vi "Update.vi"(8 "error in (no error)":errorcluster, 9 "Audio Block 2":dbl[][](array[numeric]), 10 "Audio Block 1":dbl[][](array[numeric]), 11 "Mixer in":refnum<class "Mixer.lvclass">) -> (0 "error out":errorcluster, 1 "Headphones Audio Block Out":dbl[][](array[numeric]), 2 "Master Audio Block Out":dbl[][](array[numeric]), 3 "Mixer out":refnum<class "Mixer.lvclass">)   [LabVIEW 2018, in "Mixer.lvclass"]
uses:
  Mixer.lvclass
  Mixer.lvclass/Mixer.ctl
  Channel/Channel.lvclass
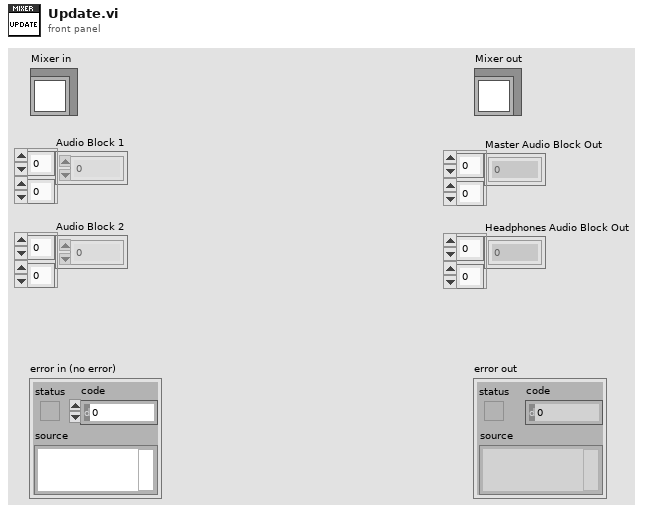
[diagram p1: front panel]
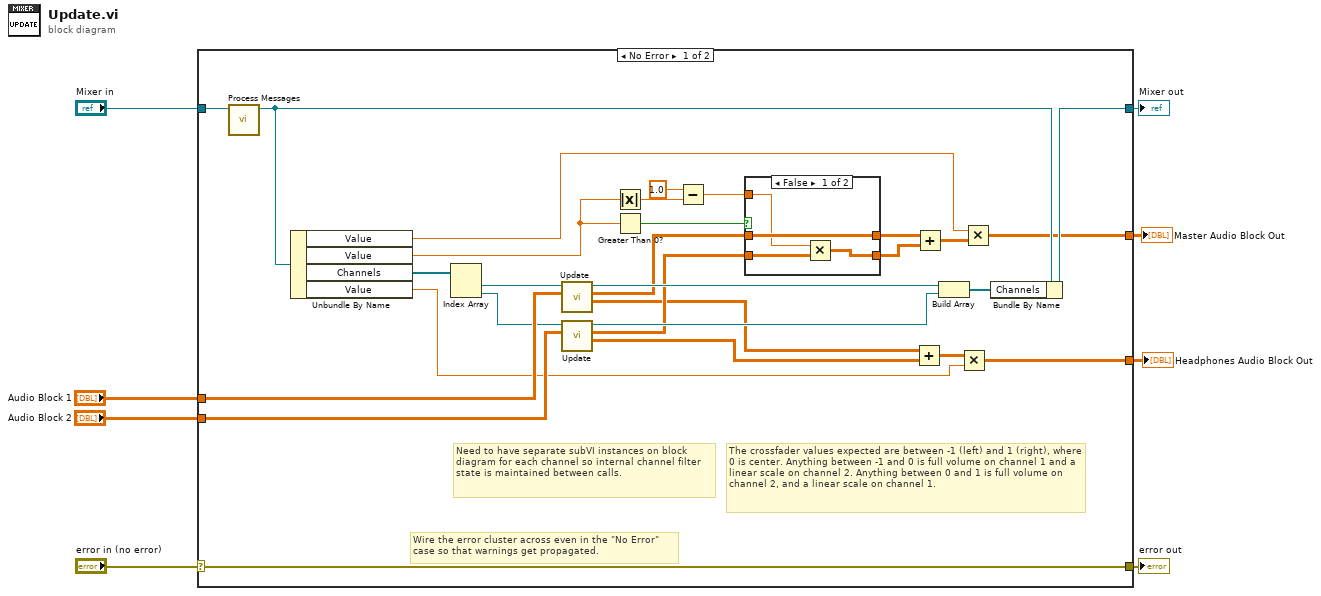
[diagram p0: block diagram]
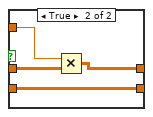
[diagram p2: hidden frame]
diagram:
  n1 = case shown="No Error" "error in (no error)" {
    selector: "error in (no error)" -> [w37 w48]
    tunnel: [w37 w48] -> w7
    tunnel: [w34 w47] -> w5
    tunnel: "Mixer in" -> [w36 w47]
    tunnel: "Audio Block 1" -> [w29 w46]
    tunnel: "Audio Block 2" -> [w28 _]
    tunnel: [w16 w46] -> w2
    tunnel: [w9 w46] -> w1
    frame No Error {
      # "Need to have separate subVI instances on block diagram for each channel so internal channel filter state is maintained between calls."
      # "The crossfader values expected are between -1 (left) and 1 (right), where 0 is center. Anything between -1 and 0 is full volume on channel 1 and a linear scale on channel 2. Anything between 0 and 1 is full volume on channel 2, and a linear scale on channel 1."
      # "Wire the error cluster across even in the \"No Error\"\ncase so that warnings get propagated."
      n2 = call "Process Messages.vi"("Mixer in"=w36) -> ("Mixer out"=w35:refnum<class "Mixer.lvclass">)  [unwired: 9 in, 1 out]
      n3 = Unbundle By Name(w35) -> ("Value"=w17:dbl, "Value"=w24:dbl, "Channels"=w33:refnum<class "Channel.lvclass">[], "Value"=w10:dbl)
      n4 = Index Array(array=w33) -> (element #1=w15:refnum<class "Channel.lvclass">, element #2=w14:refnum<class "Channel.lvclass">)  [unwired: 2 in]
      n5 = call "Update.vi"("Audio Block In"=w29, "Channel in"=w15) -> ("Headphones Audio Block Out"=w13:dbl[][], "Master Audio Block Out"=w26:dbl[][], "Channel out"=w32:refnum<class "Channel.lvclass">)  [unwired: 6 in, 1 out]
      n6 = call "Update.vi"("Audio Block In"=w28, "Channel in"=w14) -> ("Headphones Audio Block Out"=w12:dbl[][], "Master Audio Block Out"=w25:dbl[][], "Channel out"=w31:refnum<class "Channel.lvclass">)  [unwired: 6 in, 1 out]
      n7 = Absolute Value(x=w24) -> (abs(x)=w22:dbl)
      n8 = Greater Than 0?(x=w24) -> (x > 0?=w27:bool)
      n9 = Subtract(x=1.0, y=w22) -> (x-y=w21:dbl)
      n10 = case shown="False" w27 {
        tunnel: w26 -> [w39 w44]
        tunnel: w25 -> [w41 w45]
        tunnel: w21 -> [w38 w43]
        tunnel: [w40 w45] -> w19
        tunnel: [w39 w42] -> w20
        frame False {
          n11 = Multiply(x=w38, y=w41) -> (x*y=w40:dbl[][])
        }
        frame True {
          n12 = Multiply(x=w43, y=w44) -> (x*y=w42:dbl[][])
        }
      }
      n13 = Add(x=w13, y=w12) -> (x+y=w11:dbl[][])
      n14 = Add(x=w20, y=w19) -> (x+y=w18:dbl[][])
      n15 = Build Array(w32, w31) -> (w30:refnum<class "Channel.lvclass">[])
      n16 = Multiply(x=w11, y=w10) -> (x*y=w9:dbl[][])
      n17 = Multiply(x=w17, y=w18) -> (x*y=w16:dbl[][])
      n18 = Bundle By Name(cluster=w35, "Channels"=w30) -> (w34:refnum<class "Mixer.lvclass">)
    }
    frame Error {
    }
  }
  "error out" <- w7
  "Mixer out" <- w5
  "Master Audio Block Out" <- w2
  "Headphones Audio Block Out" <- w1
